vi "cross correlation test.vi"() -> ()   [LabVIEW 2012, in "Thorcam.lvclass"]
uses:
  Thorcam.lvclass
  <vilib>/vision/NI_Vision_Development_Module.lvlib
panel:
  out "System XY Graph":cluster{dbl[], dbl[]}(graph)
  out "time to calculate NCC 2":u32
  out "System Waveform Graph 2":sgl[](graph)
  in  "stop":bool
  out "error out":errorcluster
  in  "error constant":errorcluster
  in  "YOffset":i32
  in  "XOffset":i32
  out "shifted image":T1(plugin-control)
  out "original image":T1(plugin-control)
  in  "File Path to image":path
  out "crosscorrelation":T1(plugin-control)
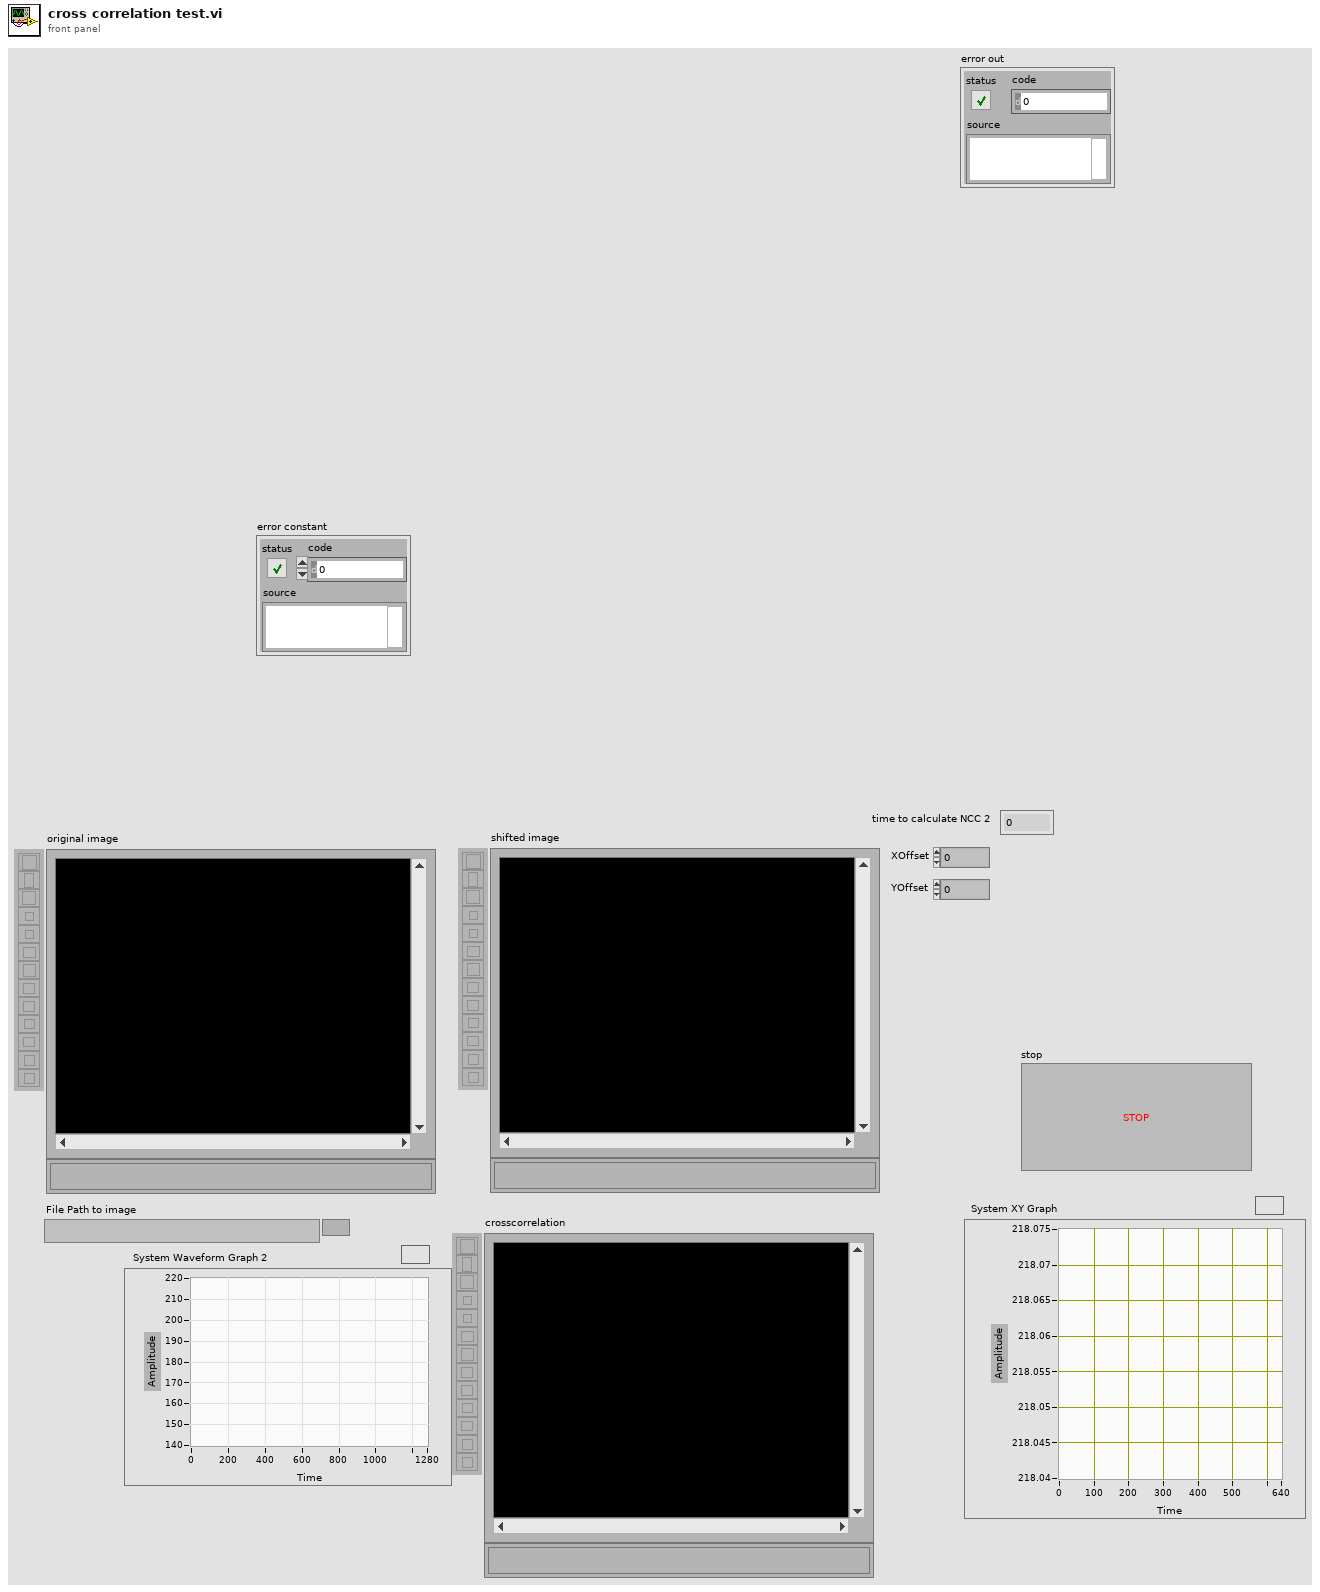
[diagram p1: front panel]
types:
  T1 = typedef "IMAQ Image.ctl" = refnum<image>
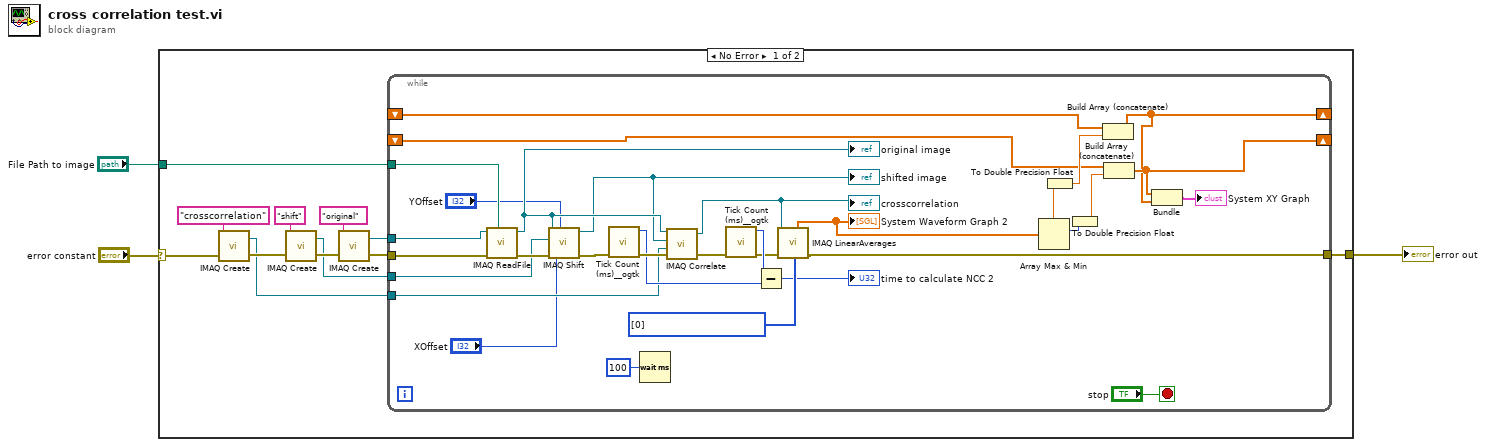
[diagram p0: block diagram]
diagram:
  n1 = case shown="No Error" "error constant" {
    selector: "error constant" -> [w8 w48]
    tunnel: "File Path to image" -> [w15 _]
    tunnel: [w14 w48] -> w1
    frame No Error {
      n2 = call "IMAQ Create"("Image Name"="crosscorrelation", "error in (no error)"=w8) -> ("New Image"=w6:T1, "error out"=w12:errorcluster)  [unwired: 3 in]
      n3 = call "IMAQ Create"("Image Name"="shift", "error in (no error)"=w12) -> ("New Image"=w5:T1, "error out"=w13:errorcluster)  [unwired: 3 in]
      n4 = call "IMAQ Create"("Image Name"="original", "error in (no error)"=w13) -> ("New Image"=w4:T1, "error out"=w7:errorcluster)  [unwired: 3 in]
      n5 = while {
        tunnel: w15 -> [w47]
        tunnel: w7 -> [w32]
        tunnel: [w38] -> w14
        tunnel: w6 -> [w31]
        tunnel: w5 -> [w30]
        tunnel: w4 -> [w29]
        shift-right: [w16] -> _
        shift-left: _ -> [w24]
        shift-right: [w17] -> _
        shift-left: _ -> [w19]
        stop <- "stop" stop-if-true
        w39 = i32[] [0] items=["X Axis Averages", "Y Axis Averages", "X + Y Axis Averages", "X - Y Axis Averages"] ("Averages")
        n6 = call "IMAQ ReadFile"("File Path"=w47, "error in (no error)"=w32, "Image"=w29) -> ("error out"=w46:errorcluster, "Image Out"=w35:T1)  [unwired: 4 in, 3 out]
        "original image" <- w35
        n7 = call "IMAQ Shift"("YOffset"="YOffset", "error in (no error)"=w46, "XOffset"="XOffset", "Image Dst"=w30, "Image Src"=w35) -> ("error out"=w45:errorcluster, "Image Dst Out"=w34:T1)  [unwired: 5 in]
        "shifted image" <- w34
        n8 = call <userlib>:"Tick Count (ms)__ogtk.vi"("error in (no error)"=w45) -> ("error out"=w44:errorcluster, "millisecond timer value"=w41:u32)  [unwired: 9 in]
        n9 = Wait (ms)(milliseconds to wait=u32 100) -> ()  [unwired: 1 out]
        n10 = call "IMAQ Correlate"("Image Src"=w35, "Image Template"=w34, "Image Dst"=w31, "error in (no error)"=w44) -> ("Image Dst Out"=w33:T1, "error out"=w43:errorcluster)  [unwired: 3 in]
        "crosscorrelation" <- w33
        n11 = call <userlib>:"Tick Count (ms)__ogtk.vi"("error in (no error)"=w43) -> ("error out"=w40:errorcluster, "millisecond timer value"=w42:u32)  [unwired: 9 in]
        n12 = Subtract(x=w42, y=w41) -> (x-y=→"time to calculate NCC 2":u32)
        n13 = call "IMAQ LinearAverages"("error in (no error)"=w40, "Averages"=w39, "Image Src"=w33) -> ("error out"=w38:errorcluster, "X Axis Averages"=w26:sgl[])  [unwired: 4 in, 3 out]
        "System Waveform Graph 2" <- w26
        n14 = Array Max & Min(array=w26) -> (max value=w22:sgl, max index (indices)=w23:i32)  [unwired: 2 out]
        n15 = To Double Precision Float(number=w22) -> (double precision float=w21:dbl)
        n16 = To Double Precision Float(number=w23) -> (double precision float=w20:dbl)
        n17 = Build Array (concatenate)(w24, w21) -> (w16:dbl[])
        n18 = Build Array (concatenate)(w19, w20) -> (w17:dbl[])
        n19 = Bundle(w17, w16) -> (→"System XY Graph":cluster{dbl[], dbl[]})  [unwired: 1 in]
      }
    }
    frame Error {
    }
  }
  "error out" <- w1
